vi "Get Manufacturer Specific Objects.vi"(8 "error in":errorcluster, 11 "reference in":refnum<class "Electronic Datasheet.lvclass">) -> (0 "error out":errorcluster, 2 "Entries":refnum<class "OD Entry.lvclass">[](array[class]), 3 "reference out":refnum<class "Electronic Datasheet.lvclass">)   [LabVIEW 2019, in "Electronic Datasheet.lvlib" / "Electronic Datasheet.lvclass"]
uses:
  Electronic Datasheet.lvclass
  Electronic Datasheet.lvclass/Electronic Datasheet.ctl
  Core/Sorted Object Dictionary/Sorted Object Dictionary.lvclass
  Core/OD Entry/OD Entry.lvclass
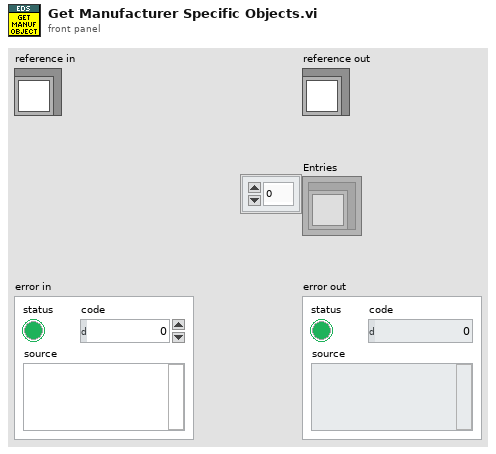
[diagram p1: front panel]
types:
  T1 = typedef "Electronic Datasheet.lvlib/Electronic Datasheet.lvclass/ObjectAttributes.ctl" = cluster{"EDS File Path":path, "Object Dict":refnum<class "Dictionary.lvclass">, "Sorted Object Dict":refnum<class "Sorted Object Dictionary.lvclass">, "Device Info":refnum<class "Device Info.lvclass">, "File Info":refnum<class "File Info.lvclass">}
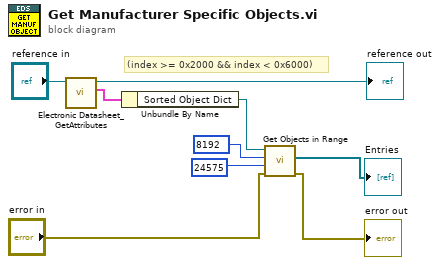
[diagram p0: block diagram]
diagram:
  # "(index >= 0x2000 && index < 0x6000)"
  n1 = call "Electronic Datasheet_GetAttributes.vi"("reference in"="reference in") -> ("Data"=w1:T1, "reference out"=→"reference out":refnum<class "Electronic Datasheet.lvclass">)  [unwired: 7 in, 2 out]
  n2 = Unbundle By Name(w1) -> ("Sorted Object Dict"=w8:refnum<class "Sorted Object Dictionary.lvclass">)
  n3 = call "Get Objects in Range.vi"("error in"="error in", "Upper Bound"=u16 24575 ("Lower Bound"), "Lower Bound"=u16 8192, "Sorted Object Dictionary in"=w8) -> ("error out"=→"error out":errorcluster, "Entries"=→"Entries":refnum<class "OD Entry.lvclass">[])  [unwired: 5 in, 1 out]
